vi "Log Inspect State Helper.vi"(7 "State Info":string, 8 "error in (no error)":errorcluster, 9 "Inspect":bool, 11 "EventLog in":refnum<class "EventLog.lvclass">) -> (0 "error out":errorcluster, 3 "EventLog out":refnum<class "EventLog.lvclass">)   [LabVIEW 2015, in "Tool Module.lvlib"]
uses:
  Tool Module.lvlib
  QC-X App/Libraries/Event Logger Library/Event Log/EventLog.lvclass
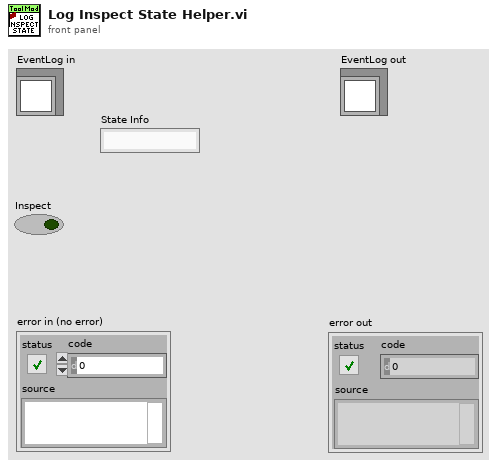
[diagram p1: front panel]
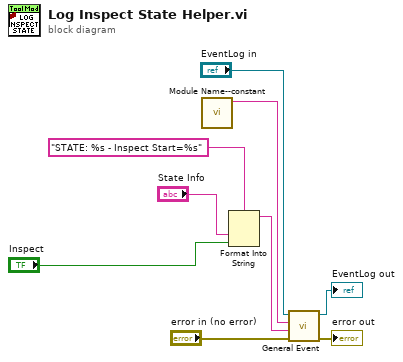
[diagram p0: block diagram]
diagram:
  n1 = call "Module Name--constant.vi"() -> ("Module Name"=w1:string)  [unwired: 11 in]
  n2 = Format Into String(format string="STATE: %s - Inspect Start=%s", "State Info", "Inspect") -> (resulting string=w8:string)  [unwired: 2 in, 1 out]
  n3 = call "General Event.vi"("error in (no error)"="error in (no error)", "Event Description"=w8, "Event Name"=w1, "EventLog ref"="EventLog in") -> ("error out"=→"error out":errorcluster, "EventLog ref"=→"EventLog out":refnum<class "EventLog.lvclass">)  [unwired: 6 in]
